vi "brians_diode_screen.vi"(0 "Diode Charts In":T1) -> ()   [LabVIEW 2017]
uses:
  diode_charts.ctl
panel:
  out "Diode Charts Out":T1={"Liquid Diodes"={1.6352471450000003, 1.7896036900000003}, "Liquid Intensity Ratio"=0.9137481969541537, "Vapor Diode"={0.0, 0.0}, "Vapor Intensity Ratio"=0.0, "TS Window 1 Temperatures"={"Average"=21.026813909635873, "T Sat [C]"=13.792788916308993}}
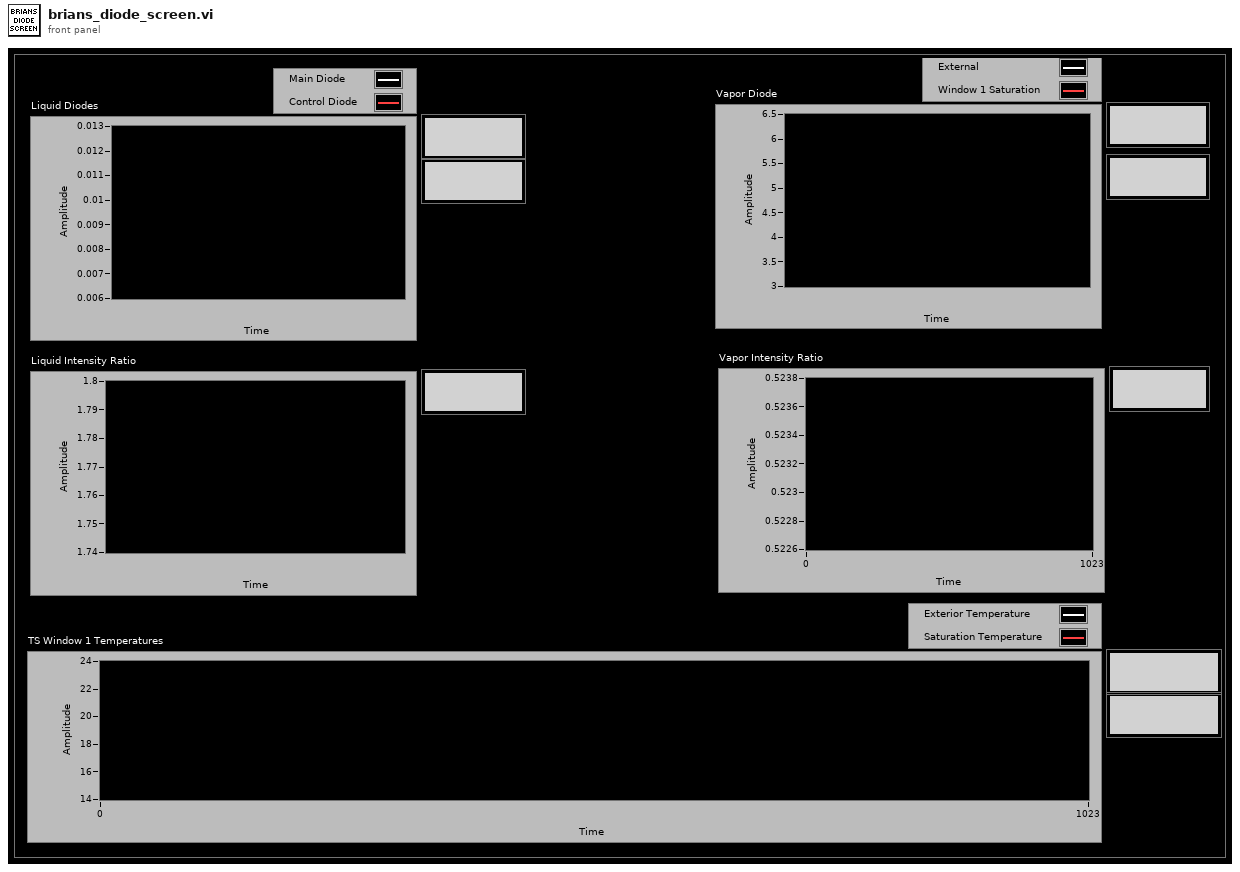
[diagram p1: front panel]
types:
  T1 = typedef "diode_charts.ctl" = cluster{"Liquid Diodes":cluster{dbl, dbl}, "Liquid Intensity Ratio":dbl, "Vapor Diode":cluster{dbl, dbl}, "Vapor Intensity Ratio":dbl, "TS Window 1 Temperatures":cluster{"Average":dbl, "T Sat [C]":dbl}}
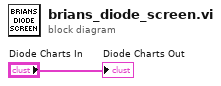
[diagram p0: block diagram]
diagram:
  "Diode Charts Out" <- "Diode Charts In"
